vi "OAT Remove Extra Boundaries.vi"(5 "RPM indices in":i32[](array[numeric]), 7 "time of RPM boundaries in":i32[](array[numeric])) -> (1 "RPM indices out":i32[](array[numeric]), 3 "time of RPM boundaries out":i32[](array[numeric]))   [LabVIEW 2017, in "SoundVib_Gabor.lvlib"]
uses:
  <vilib>/addons/Sound and Vibration/Order Analysis/Gabor Order Tracking/SoundVib_Gabor.lvlib
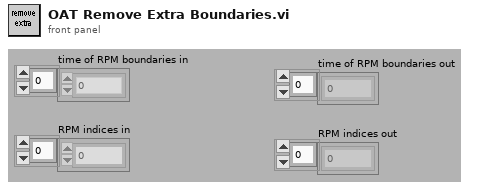
[diagram p1: front panel]
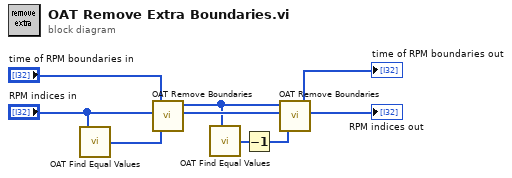
[diagram p0: block diagram]
diagram:
  n1 = call <vilib>:"OAT Find Equal Values.vi"("array in"="RPM indices in") -> ("equal indices"=w9:i32[])
  n2 = call <vilib>:"OAT Remove Boundaries.vi"("indices to remove"=w9, "array 2 in"="RPM indices in", "array 1 in"="time of RPM boundaries in") -> ("array 2 out"=w4:i32[], "array 1 out"=w2:i32[])  [unwired: 3 in]
  n3 = call <vilib>:"OAT Find Equal Values.vi"("array in"=w2) -> ("equal indices"=w8:i32[])
  n4 = Decrement(x=w8) -> (x-1=w3:i32[])
  n5 = call <vilib>:"OAT Remove Boundaries.vi"("indices to remove"=w3, "array 2 in"=w4, "array 1 in"=w2) -> ("array 2 out"=→"RPM indices out":i32[], "array 1 out"=→"time of RPM boundaries out":i32[])  [unwired: 3 in]
